vi "HeaderAction.vi"(0 "EG_G5210 en entrée":refnum<class "EG_G5210.lvclass"> caption="DNL_LabVIEW Object in", 11 "error in (no error)":errorcluster caption="entrée d'erreur (pas d'erreur)") -> (4 "EG_G5210 en sortie":refnum<class "EG_G5210.lvclass"> caption="DNL_LabVIEW Object out", 6 "DataNames":string[](array[string]), 8 "Instr Name":string, 10 "HeaderString":string, 15 "error out":errorcluster caption="sortie d'erreur")   [LabVIEW 2010, in "EG_G5210.lvclass"]
uses:
  EG_G5210.lvclass
  EG_G5210.lvclass/EG_G5210.ctl
  BaseDevice/BaseDevice.lvclass
  <userlib>/EG_G 5210 LIA/ReadFunctions.ctl
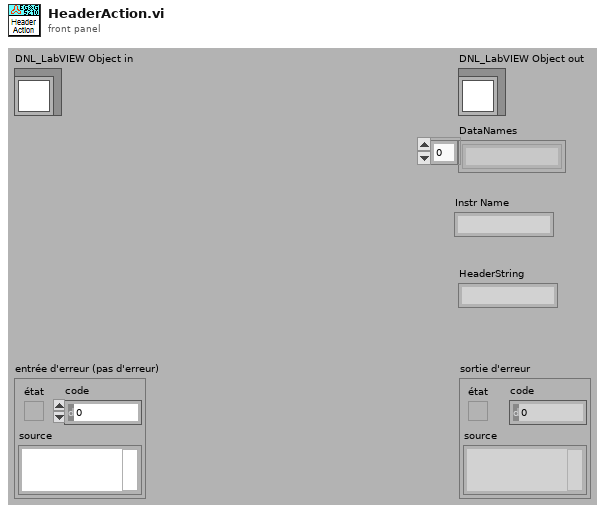
[diagram p1: front panel]
types:
  T1 = typedef "ReadFunctions.ctl" = enum16{"Sensitivity", "Vernier Mode", "Main Filter", "Filter Mode", "Line Filter", "Ref Source", "Ref Mode", "Ref Phase", "Ref Frequency", "Output Filter", "Time Constant", "Dyn Reserve", "X Offset", "Y Offset", "Expand Mode", "Int Oscillator", "Oscillator Freq", "All params", "Overload Byte", "Trigger Mode", "Error"}
  T2 = typedef "EG_G5210.lvclass/EG_G5210_Func.ctl" = enum16{"Read X & Y (V)", "Read Mag & Phase (V,°)", "Read X, Y, Mag & Phase (V,V,V,°)", "Read ADC Ch1 (V)", "Read ADC Ch2 (V)"}
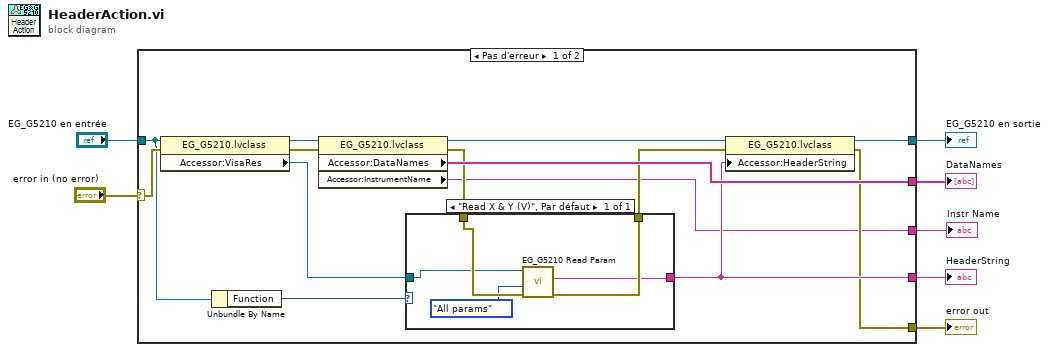
[diagram p0: block diagram]
diagram:
  n1 = case shown="Pas d'erreur" "error in (no error)" {
    selector: "error in (no error)" -> [w18 w27]
    tunnel: "EG_G5210 en entrée" -> [w10 w28]
    tunnel: [w14 w28] -> w5
    tunnel: [w20 _] -> w4
    tunnel: [w13 _] -> w3
    tunnel: [w11 w27] -> w2
    tunnel: [w8 _] -> w1
    frame No Error {
      n2 = property class="EG_G5210.lvclass"(reference=w10, error in=w18) -> (reference out=w19:refnum<class "EG_G5210.lvclass">, error out=w16:errorcluster, "Accessor:VisaRes"=w17:refnum<visa-resource-name>)
      n3 = Unbundle By Name(w10) -> ("Function"=w9:T2)
      n4 = property class="EG_G5210.lvclass"(reference=w19, error in=w16) -> (reference out=w21:refnum<class "EG_G5210.lvclass">, error out=w15:errorcluster, "Accessor:DataNames"=w20:string[], "Accessor:InstrumentName"=w8:string)
      n5 = case shown="\"Read X & Y (V)\", Par défaut" w9 {
        tunnel: w17 -> [w24]
        tunnel: w15 -> [w26]
        tunnel: [w23] -> w13
        tunnel: [w25] -> w12
        frame "Read X & Y (V)", Default {
          n6 = call <userlib>:"EG_G5210 Read Param.vi"("error in (no error)"=w26, "Énum"=ReadFunctions."All params", "Ressource VISA"=w24) -> ("error out"=w25:errorcluster, "Params"=w23:string)  [unwired: 5 in, 2 out]
        }
      }
      n7 = property class="EG_G5210.lvclass"(reference=w21, error in=w12, "Accessor:HeaderString"=w13) -> (reference out=w14:refnum<class "EG_G5210.lvclass">, error out=w11:errorcluster)
    }
    frame Error {
    }
  }
  "error out" <- w2
  "EG_G5210 en sortie" <- w5
  "DataNames" <- w4
  "HeaderString" <- w3
  "Instr Name" <- w1
